vi "Handle Error.vi"(8 "error in (no error)":errorcluster, 11 "CS++DeviceActor in":refnum<class "CS++DeviceActor.lvclass">) -> (0 "error out":errorcluster, 2 "stop actor?":bool=TRUE, 3 "CS++DeviceActor out":refnum<class "CS++DeviceActor.lvclass">)   [LabVIEW 2012, in "CS++DeviceActor.lvlib" / "CS++DeviceActor.lvclass"]
doc: "(<B>Filename</B>: Actor Framework.lvlib:Actor.lvclass:Handle Error.vi)\n\nDefines how the actor handles an error that occurred while processing a message.\n\nBy default, this method does nothing except stop the actor. This method also treats error code 43 (coming from <B>error in</B>) as a sign that the actor shut down normally. In this situation, the Handle Error method does not return the error on <B>error out</B>, meaning the actor's caller will not receive it. All other error codes will be returned on <B>error out</B>.\n\nA descendant class may override this method to change this behavior."
uses:
  CS++DeviceActor.lvclass
  CS++Reservable/CS++ReservableActor.lvclass
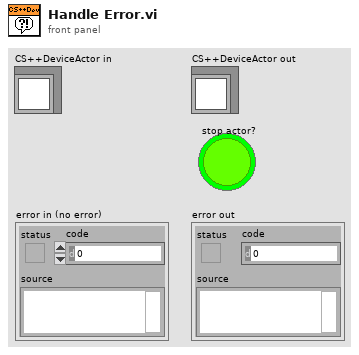
[diagram p1: front panel]
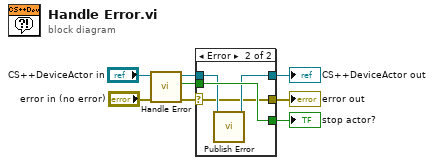
[diagram p0: block diagram]
diagram:
  n1 = call-parent "Handle Error.vi"("error in (no error)"="error in (no error)", "CS++BaseActor in"="CS++DeviceActor in") -> ("error out"=w4:errorcluster, "stop actor?"=w5:bool, "CS++BaseActor out"=w6:refnum<class "CS++DeviceActor.lvclass">)  [unwired: 7 in]
  n2 = case shown="Error" w4 {
    selector: w4 -> [w11 w12]
    tunnel: [w11 w12] -> w1
    tunnel: [w10 w15] -> w2
    tunnel: w5 -> [w10 w15]
    tunnel: [w9 w13] -> w3
    tunnel: w6 -> [w9 w14]
    frame No Error {
    }
    frame Error {
      n3 = call "Publish Error.vi"("CS++DeviceActor in"=w14) -> ("CS++DeviceActor out"=w13:refnum<class "CS++DeviceActor.lvclass">)  [unwired: 9 in, 1 out]
    }
  }
  "CS++DeviceActor out" <- w3
  "error out" <- w1
  "stop actor?" <- w2
